vi "Read(LIST).vi"(8 "error in (no error)":errorcluster, 10 "Spot No.":i32=1 min=1 max=10 step=1, 11 "VISA resource name":refnum<visa-resource-name>) -> (0 "error out":errorcluster, 1 "Secondary Value":dbl, 2 "Primary Value":dbl, 3 "VISA resource name out":refnum<visa-resource-name>, 4 "COMP Result":string, 5 "Spot No.":i32)   [LabVIEW 2014, in "LCR Meter.lvlib"]
doc: "Query the latest LIST measurement data of the primary parameters, secondary parameters and comparator results into the output buffer.\n\n<B>Note</B>\nOnly applicable when in the [LIST MEAS] page view."
uses:
  <instrlib>/LCR Meter/Examples/LCR Meter Acquire Single_1 Folder/LCR Meter.lvlib
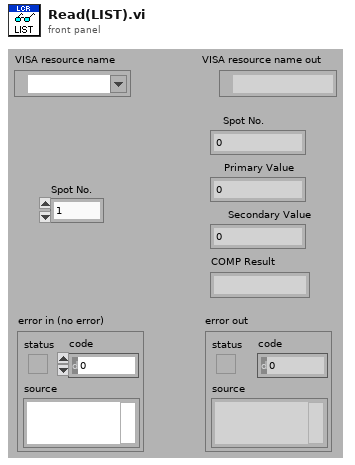
[diagram p1: front panel]
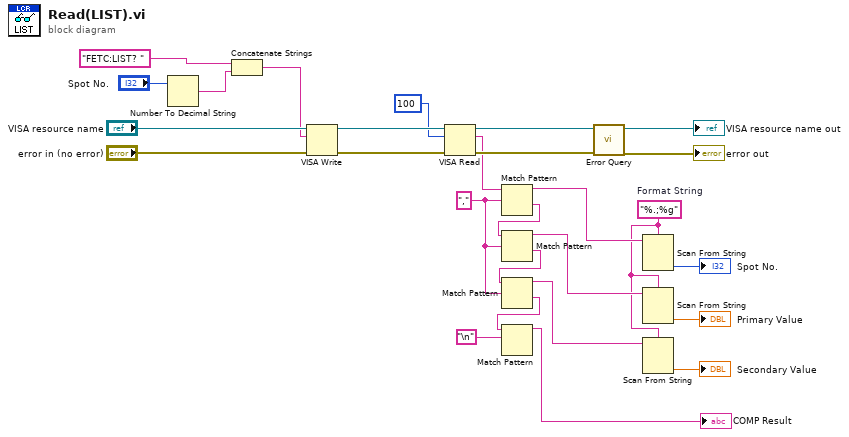
[diagram p0: block diagram]
diagram:
  w5 = "%.;%g"  # Format String
  w6 = "," ("regular expression")
  n1 = Number To Decimal String(number="Spot No.") -> (decimal integer string=w21:string)  [unwired: 1 in]
  n2 = Concatenate Strings("FETC:LIST? ", w21) -> (w20:string)
  n3 = VISA Write(VISA resource name="VISA resource name", write buffer=w20, error in (no error)="error in (no error)") -> (VISA resource name out=w19:refnum<visa-resource-name>, error out=w18:errorcluster)  [unwired: 1 out]
  n4 = VISA Read(VISA resource name=w19, byte count=u32 100, error in (no error)=w18) -> (VISA resource name out=w17:refnum<visa-resource-name>, read buffer=w1:string, error out=w16:errorcluster)  [unwired: 1 out]
  n5 = Match Pattern(string=w1, regular expression=w6) -> (before substring=w12:string, after substring=w9:string)  [unwired: 1 in, 2 out]
  n6 = Match Pattern(string=w9, regular expression=w6) -> (before substring=w11:string, after substring=w10:string)  [unwired: 1 in, 2 out]
  n7 = Match Pattern(string=w10, regular expression=w6) -> (before substring=w4:string, after substring=w7:string)  [unwired: 1 in, 2 out]
  n8 = Match Pattern(string=w7, regular expression="\n") -> (before substring=→"COMP Result":string)  [unwired: 1 in, 3 out]
  n9 = call <instrlib>:"Error Query.vi"("error in (no error)"=w16, "VISA resource name"=w17) -> ("error out"=→"error out":errorcluster, "VISA resource name out"=→"VISA resource name out":refnum<visa-resource-name>)  [unwired: 6 in, 2 out]
  n10 = Scan From String(format string=w5, input string=w12) -> (output 1=→"Spot No.":i32)  [unwired: 3 in, 3 out]
  n11 = Scan From String(format string=w5, input string=w11) -> (output 1=→"Primary Value":dbl)  [unwired: 3 in, 3 out]
  n12 = Scan From String(format string=w5, input string=w4) -> (output 1=→"Secondary Value":dbl)  [unwired: 3 in, 3 out]
